vi "List Polymorphic.vi"   [LabVIEW 2020, in "NI_VIAnCFGDataStructure.lvlib" / "Tree.lvclass"]
doc: "Polymorphic instance of the List method. Select the appropraite instance to work with or allow this method to adapt automatically."
uses:
  <vilib>/addons/analyzer/VIAnCFGDataStructure/Tree Manager/Tree.lvclass
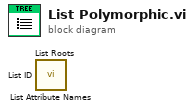
[diagram p0: block diagram]
diagram:
  n1 = call <vilib>:"List Attribute Names.vi"() -> ()  [unwired: 9 in, 3 out]
  n2 = call <vilib>:"List Roots.vi"() -> ()  [unwired: 8 in, 4 out]
  n3 = call <vilib>:"List ID.vi"() -> ()  [unwired: 8 in, 4 out]
